vi "GodlewskiPiotr-Zad2.vi"() -> ()   [LabVIEW 2020]
panel:
  out "MIN temp":dbl
  out "MAX temp":dbl
  in  "N":i32=100
  out "T œrednie":dbl
  out "T chwilowe":dbl
  out "Alarm górny":bool
  out "Alarm dolny":bool
  in  "Próg górny":dbl=25.8
  in  "Próg dolny":dbl
  in  "Zapis do pliku":bool
  in  "URL":string="dstp://192.168.159.1/temperatura"
  in  "stop":bool
  out "Temperatura":T1(graph)
  # "Zadanie dodatkowe 1"
  # "Wartoœæ maksymalna i minimalna z N ostatnich próbek"
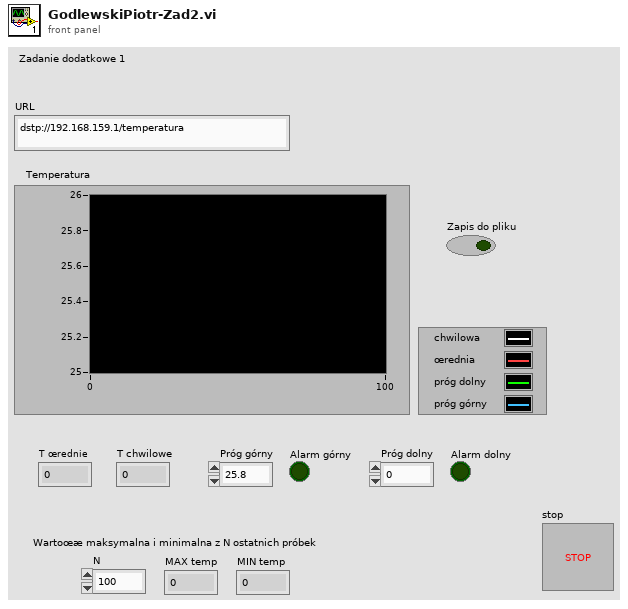
[diagram p1: front panel]
types:
  T1 = cluster{dbl, dbl, "Próg dolny":dbl, "Próg górny":dbl}
  T2 = enum16{"Read", "Write", "ReadWrite", "BufferedRead", "BufferedReadWrite"}
  T3 = enum16{"open", "replace", "create", "open or create", "replace or create", "replace or create with confirmation"}
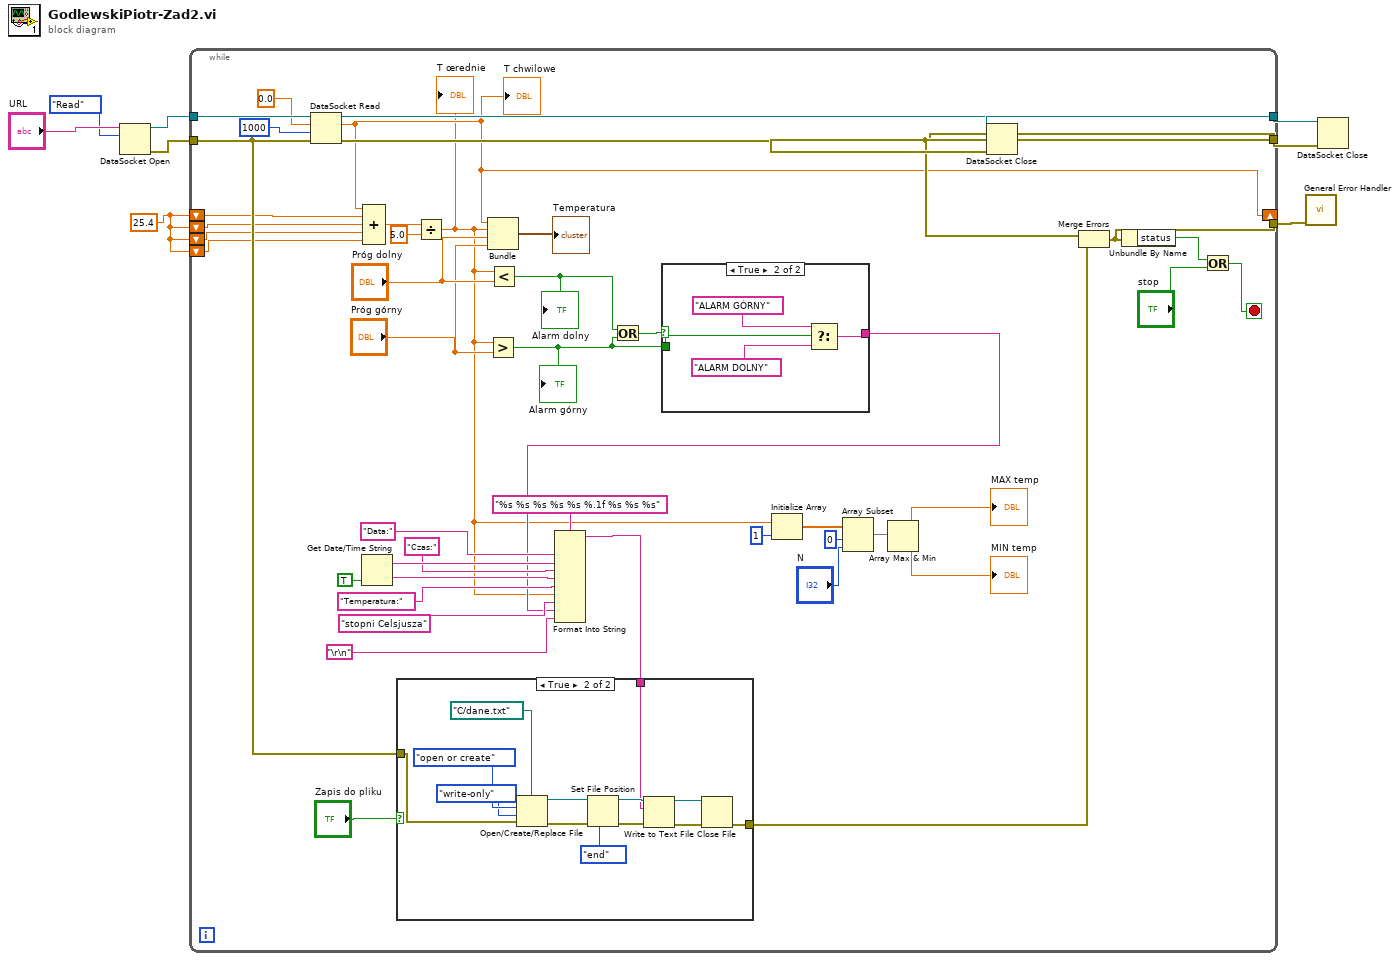
[diagram p0: block diagram]
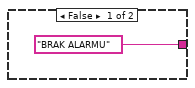
[diagram p2: hidden frame]
diagram:
  w1 = 25.4
  n1 = DataSocket Open(10:T2."Read" ("mode"), 11:"URL") -> (0:w7:errorcluster, 3:w8:refnum<k13>)  [unwired: 2 in]
  n2 = while {
    tunnel: w8 -> [w51]
    tunnel: [w50] -> w3
    tunnel: w7 -> [w44]
    tunnel: [w22] -> w2
    tunnel: [w42] -> w5
    shift-right: [w17] -> _
    shift-left: w1 -> [w21]
    shift-left: w1 -> [w20]
    shift-left: w1 -> [w19]
    shift-left: w1 -> [w18]
    stop <- w48 stop-if-true
    n3 = DataSocket Read(8:w44, 9:1000, 10:0.0, 11:w51) -> (0:w22:errorcluster, 2:w17:dbl, 3:w50:refnum<k13>)  [unwired: 1 in, 4 out]
    "T chwilowe" <- w17
    n4 = Get Date/Time String(want seconds? (F)=TRUE) -> (date string=w39:string, time string=w37:string)  [unwired: 2 in]
    n5 = Compound Arithmetic op=ADD(w17, w21, w20, w19, w18) -> (w31:dbl)
    n6 = Divide(x=w31, y=5.0 ("x/y")) -> (x/y=w11:dbl)
    "T œrednie" <- w11
    n7 = Bundle(w17, w11, "Próg dolny"="Próg dolny", "Próg górny"="Próg górny") -> (→"Temperatura":T1)  [unwired: 1 in]
    n8 = Greater?(x=w11, y="Próg górny") -> (0:w24:bool)
    "Alarm górny" <- w24
    n9 = Less?(x=w11, y="Próg dolny") -> (x < y?=w27:bool)
    "Alarm dolny" <- w27
    n10 = Or(x=w27, y=w24) -> (x .or. y?=w26:bool)
    n11 = case shown="True" w26 {
      tunnel: ["BRAK ALARMU" w55] -> w25
      tunnel: w24 -> [_ w54]
      frame False {
      }
      frame True {
        n12 = Select(t="ALARM GÓRNY", s=w54, f="ALARM DOLNY") -> (s? t:f=w55:string)
      }
    }
    n13 = Format Into String(format string="%s %s %s %s %s %.1f %s %s %s", "Data:", w39, "Czas:", w37, "Temperatura:", w11, "stopni Celsjusza", w25, "\r\n") -> (resulting string=w23:string)  [unwired: 2 in, 1 out]
    n14 = case shown="True" "Zapis do pliku" {
      tunnel: w44 -> [w58 w66]
      tunnel: [w58 w62] -> w43
      tunnel: w23 -> [_ w59]
      frame False {
      }
      frame True {
        n15 = Open/Create/Replace File(file path (use dialog)=path "C:/dane.txt", error in=w66, operation (0:open)=T3."open or create", access (0:read/write)=enum16{"read/write", "read-only", "write-only"}."write-only") -> (refnum out=w64:refnum<file>, error out=w65:errorcluster)  [unwired: 2 in, 1 out]
        n16 = Set File Position(refnum=w64, from (0:start)=enum16{"start", "end", "current"}."end", error in=w65) -> (refnum out=w67:refnum<file>, error out=w68:errorcluster)  [unwired: 1 in]
        n17 = Write to Text File(file (use dialog)=w67, text=w59, error in=w68) -> (refnum out=w69:refnum<file>, error out=w70:errorcluster)  [unwired: 1 in, 1 out]
        n18 = Close File(refnum=w69, error in=w70) -> (error out=w62:errorcluster)  [unwired: 1 out]
      }
    }
    n19 = Initialize Array(w11, 1 ("dimension size")) -> (w13:dbl[])
    n20 = Array Subset(array=w13, index=0, length="N") -> (w12:dbl[])
    n21 = Array Max & Min(array=w12) -> (max value=→"MAX temp":dbl, min value=→"MIN temp":dbl)  [unwired: 2 out]
    n22 = Merge Errors(w22, w43) -> (w42:errorcluster)
    n23 = Unbundle By Name(w42) -> ("status"=w49:bool)
    n24 = Or(x=w49, y="stop") -> (x .or. y?=w48:bool)
  }
  n25 = DataSocket Close(8:w2, 11:w3) -> ()  [unwired: 1 in, 2 out]
  n26 = call <vilib>:"General Error Handler.vi"("error in (no error)"=w5) -> ()  [unwired: 10 in, 5 out]
  n27 = DataSocket Close(8:w2, 11:w3) -> ()  [unwired: 1 in, 2 out]
